vi "dataUnpackBoolArray.vi"(8 "errorIn":errorcluster, 11 "data":variant) -> (0 "errorOut":errorcluster, 3 "boolArray":bool[](array[boolean]))   [LabVIEW 2017]
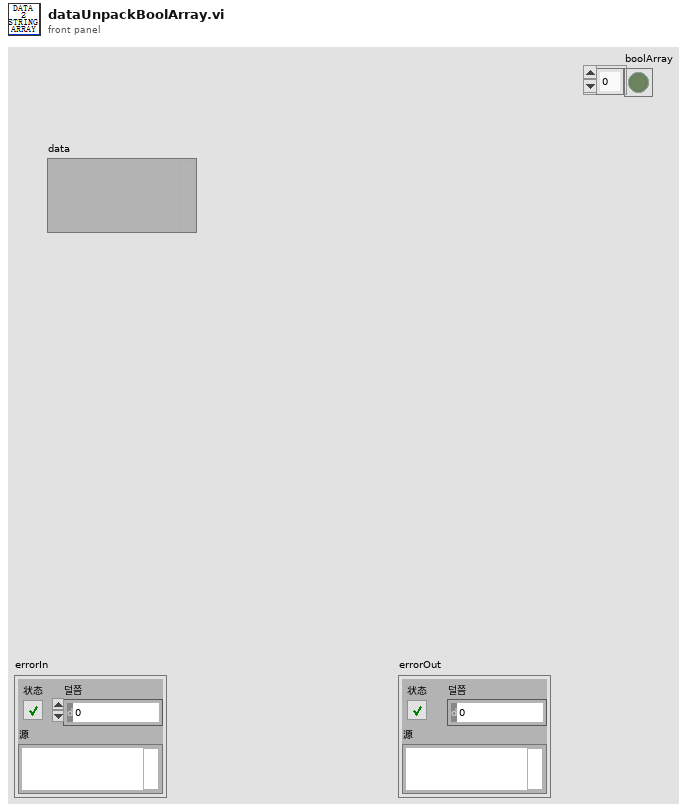
[diagram p1: front panel]
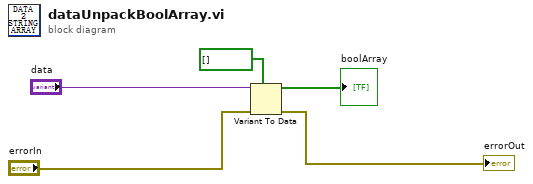
[diagram p0: block diagram]
diagram:
  n1 = Variant To Data(error in="errorIn", type=bool[] [], Variant="data") -> (data=→"boolArray":bool[], error out=→"errorOut":errorcluster)
